vi "Print Initialization Message.vi"(8 "error in (no error)":errorcluster, 11 "Parameters":T1={"Interface Data"={"Name"="", "Unit ID"=0, "Refresh Rate"=0, "Write Rate"=0, "Write Mode"=enum."Value Change", "Interface Type"=enum."TCP Master", "TCP Settings"={"Address"="", "Port"=0, "Timeout"=0}, "Serial Settings"={"VISA resource name"="", "baud rate"=0, "parity (even)"=0, "flow control (none)"=0, "serial type"=enum."RTU", "Wire Mode"=-1}}, "Modbus Input Groups"=[], "Modbus Output Groups"=[], "error in (no error)"={"status"=FALSE, "code"=0, "source"=""}, "Modbus Input Engine Group Names"=[], "Modbus Output Engine Group Names"=[]} {"Interface Data"."Serial Settings"."Wire Mode" items=["Unknown"=-1, "RS485/Wire4"=0, "RS485/Wire2-EchoDTR"=1, "RS485/Wire2-CtrlDTR"=2, "RS485/Wire2-Auto"=3, "RS232/DTE"=128, "RS232/DCE"=129, "RS232/AUTO"=130]; "Interface Data"."Serial Settings"."parity (even)" items=["None", "Odd", "Even", "Mark", "Space"]; "Interface Data"."Serial Settings"."flow control (none)" items=["None", "XON/XOFF", "RTS/CTS", "XON/XOFF & RTS/CTS", "DTR/DSR", "XON/XOFF & DTR/DSR"]}) -> (0 "error out":errorcluster)   [LabVIEW 2020, in "Modbus Master Engine.lvlib"]
uses:
  Modbus Master Engine.lvlib
  Shared/Device Info.ctl
  Shared/Write Mode.ctl
  Shared/Controls/Interface Type.ctl
  Shared/Controls/Data Model/TCP Settings.ctl
  Shared/Controls/Data Model/Serial Settings.ctl
  Bulk Data Access.ctl
  System Explorer/SubVIs/Modbus Type.ctl
  Shared/Controls/Data Model/Channel.ctl
  <vilib>/NI VeriStand/Custom Device API/Custom Device Channel Type.ctl
  Shared/Controls/Data Model/Mapping.ctl
  Shared/Controls/Data Model/DataType.ctl
  <vilib>/NI VeriStand/Custom Device API/Custom Device Item Ref.ctl
  <vilib>/NI VeriStand/Custom Device Tools/Custom Device Utility Library/Custom Device Utility Library.lvlib
  Shared/Modbus Master Shared.lvlib
  <vilib>/NI VeriStand/Custom Device API/Custom Device API.lvlib
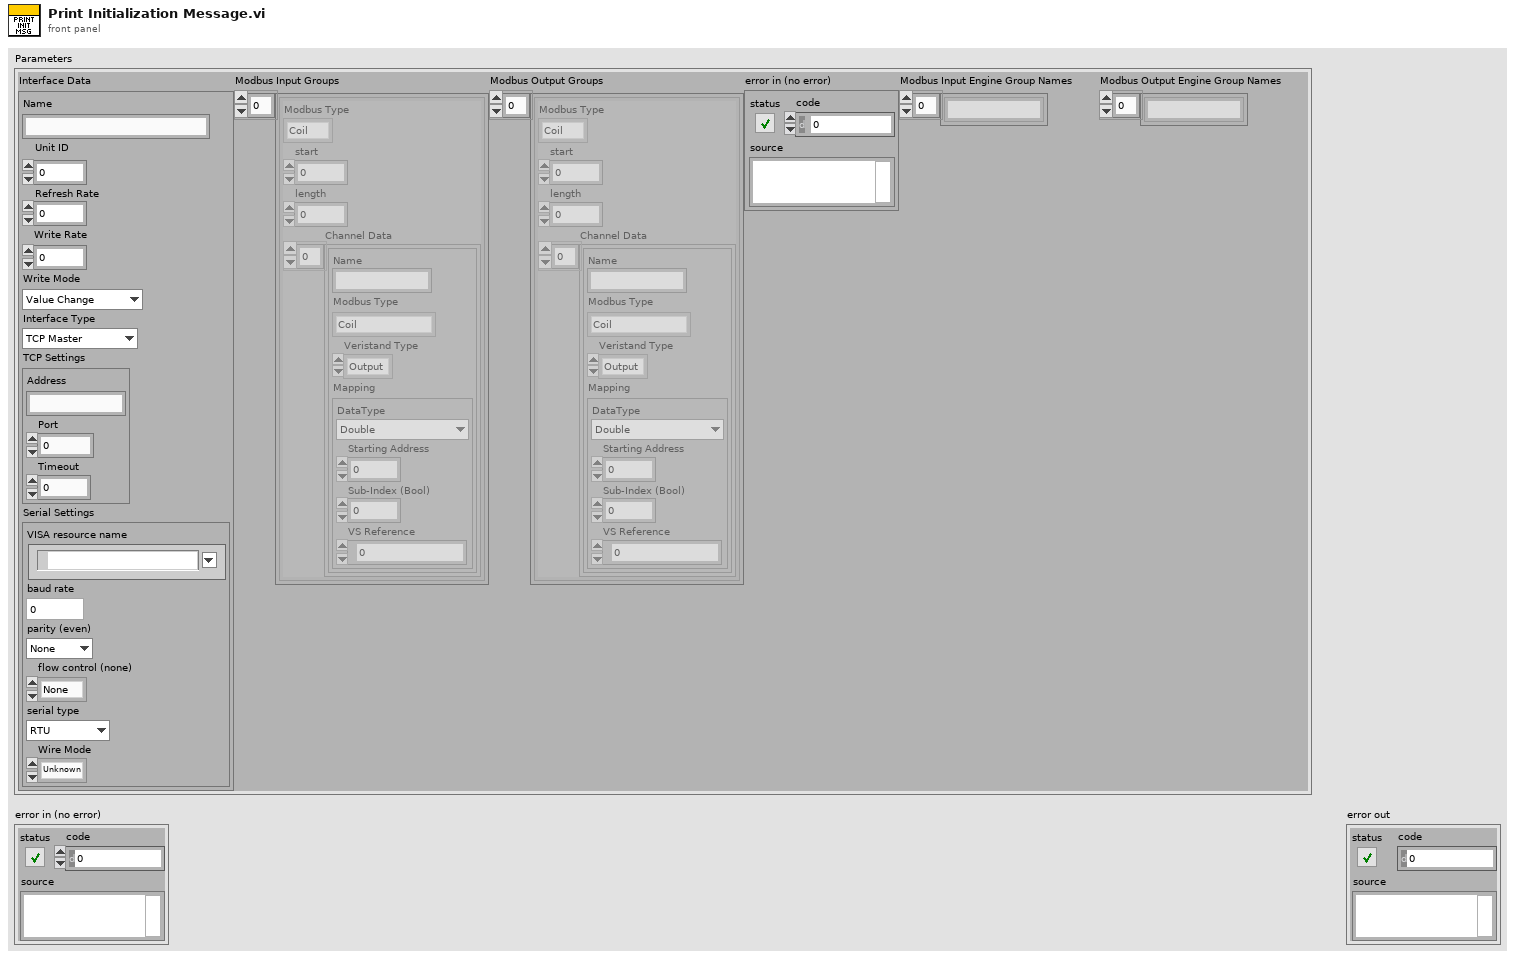
[diagram p1: front panel]
types:
  T1 = typedef "Modbus Master Shared.lvlib/Device Info.ctl" = cluster{"Interface Data":cluster{"Name":string, "Unit ID":u8, "Refresh Rate":i32, "Write Rate":i32, "Write Mode":T2, "Interface Type":T3, "TCP Settings":T4, "Serial Settings":T5}, "Modbus Input Groups":T6[], "Modbus Output Groups":T6[], "error in (no error)":errorcluster, "Modbus Input Engine Group Names":string[], "Modbus Output Engine Group Names":string[]}
  T2 = typedef "Modbus Master Shared.lvlib/Write Mode.ctl" = enum16{"Value Change", "Interval"}
  T3 = typedef "Modbus Master Shared.lvlib/Interface Type.ctl" = enum16{"TCP Master", "Serial Master", "TCP Slave", "Serial Slave"}
  T4 = typedef "Modbus Master Shared.lvlib/TCP Settings.ctl" = cluster{"Address":string, "Port":u16, "Timeout":i32}
  T5 = typedef "Modbus Master Shared.lvlib/Serial Settings.ctl" = cluster{"VISA resource name":refnum<visa-resource-name>, "baud rate":u32, "parity (even)":u16, "flow control (none)":u16, "serial type":enum16{"RTU", "ASCII"}, "Wire Mode":i16}
  T6 = typedef "Modbus Master Shared.lvlib/Bulk Data Access.ctl" = cluster{"Modbus Type":T7, "start":u16, "length":u16, "Channel Data":T8[]}
  T7 = typedef "Modbus Master Shared.lvlib/Modbus Type.ctl" = enum16{"Coil", "Discrete Input", "Holding Register", "Input Register"}
  T8 = typedef "Modbus Master Shared.lvlib/Channel.ctl" = cluster{"Name":string, "Modbus Type":T7, "Veristand Type":T9, "Mapping":T10}
  T9 = typedef "Custom Device API.lvlib/Custom Device Channel Type.ctl" = enum16{"Input", "Output"}
  T10 = typedef "Modbus Master Shared.lvlib/Mapping.ctl" = cluster{"DataType":T11, "Starting Address":u16, "Sub-Index (Bool)":u16, "VS Reference":T12}
  T11 = typedef "Modbus Master Shared.lvlib/DataType.ctl" = enum16{"Double", "Single", "I64", "I32", "I16", "I8", "U64", "U32", "U16", "U8", "Boolean"}
  T12 = typedef "Custom Device API.lvlib/Custom Device Item Ref.ctl" = u64
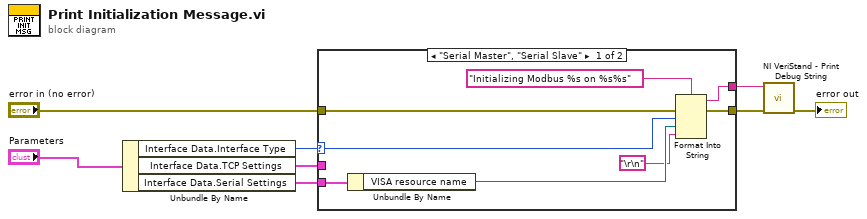
[diagram p0: block diagram]
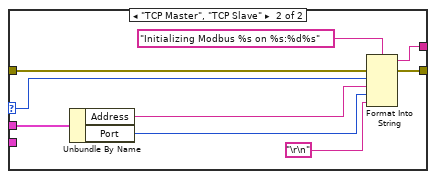
[diagram p2: hidden frame]
diagram:
  n1 = Unbundle By Name("Parameters") -> ("Interface Data.Interface Type"=w5:T3, "Interface Data.TCP Settings"=w7:T4, "Interface Data.Serial Settings"=w6:T5)
  n2 = case shown="\"Serial Master\", \"Serial Slave\"" w5 {
    selector: w5 -> [w15 w24]
    tunnel: w6 -> [w14 _]
    tunnel: w7 -> [_ w22]
    tunnel: "error in (no error)" -> [w12 w20]
    tunnel: [w11 w19] -> w2
    tunnel: [w10 w18] -> w3
    frame "Serial Master", "Serial Slave" {
      n3 = Unbundle By Name(w14) -> ("VISA resource name"=w13:refnum<visa-resource-name>)
      n4 = Format Into String(format string="Initializing Modbus %s on %s%s", error in=w12, w15, w13, "\r\n") -> (resulting string=w10:string, error out=w11:errorcluster)  [unwired: 1 in]
    }
    frame "TCP Master", "TCP Slave" {
      n5 = Unbundle By Name(w22) -> ("Address"=w23:string, "Port"=w21:u16)
      n6 = Format Into String(format string="Initializing Modbus %s on %s:%d%s", error in=w20, w24, w23, w21, "\r\n") -> (resulting string=w18:string, error out=w19:errorcluster)  [unwired: 1 in]
    }
  }
  n7 = call <vilib>:"NI VeriStand - Print Debug String.vi"("error in (no error)"=w2, "Message"=w3) -> ("error out"=→"error out":errorcluster)  [unwired: 9 in]
